vi "ProjectionExp_B.vi"() -> ()   [LabVIEW 2017]
uses:
  <instrlib>/Tektronix TDS 200 1000 2000 Series/Tektronix TDS 200 1000 2000 Series.lvlib
panel:
  in  "p":dbl
  out "Backgrond Light Intensity":dbl
  out "Units 2":string
  out "error out 3":errorcluster
  in  "Resource Name for Background":refnum<visa-resource-name>
  in  "Channel (1: Channel 1) 2":i32(ring)=1 items=["Channel 1"=1, "Channel 2"=2, "Channel 3"=3, "Channel 4"=4]
  in  "Background Light Intensity Type":i32(ring) items=["Frequency", "Mean", "Period", "Pulse Duty", "Peak to Peak", "Cycle RMS", "Minimum", "Maximum", "Rise Time", "Fall Time", "Positive Width", "Negative Width", "Amplitude", "Cycle Mean", "High", "Low", "Negative Duty", "Positive Overshoot", "Negative Overshoot", "Cursor Mean", "Burst Width", "Positive Pulse Count", "Negative Pulse Count", "Rising Edge Count", "Falling Edge Count", "Area", "Cycle Area", "RMS", "Cursor RMS"]
  in  "error in (no error) 3":errorcluster
  out "error out 2":errorcluster caption="error out"
  in  "Delay Time (s)":dbl=1.0
  in  "error in (no error) 2":errorcluster caption="error in (no error)"
  out "Iteration":i32
  out "Phi":dbl[][](array[numeric])
  out "y (Measurement \nMatrix)":dbl[][](array[numeric])
  out "VISA resource name out":refnum<visa-resource-name>
  out "Measurement":dbl
  out "Units":string
  out "error out":errorcluster
  in  "VISA resource name":refnum<visa-resource-name>
  in  "Channel (1: Channel 1)":i32(ring)=1 items=["Channel 1"=1, "Channel 2"=2, "Channel 3"=3, "Channel 4"=4]
  in  "Measurement Type (0: Frequency)":i32(ring) items=["Frequency", "Mean", "Period", "Pulse Duty", "Peak to Peak", "Cycle RMS", "Minimum", "Maximum", "Rise Time", "Fall Time", "Positive Width", "Negative Width", "Amplitude", "Cycle Mean", "High", "Low", "Negative Duty", "Positive Overshoot", "Negative Overshoot", "Cursor Mean", "Burst Width", "Positive Pulse Count", "Negative Pulse Count", "Rising Edge Count", "Falling Edge Count", "Area", "Cycle Area", "RMS", "Cursor RMS"]
  in  "error in (no error)":errorcluster
  out "Theta":dbl[][](array[numeric])
  in  "k":dbl
  in  "m":dbl
  in  "n":dbl
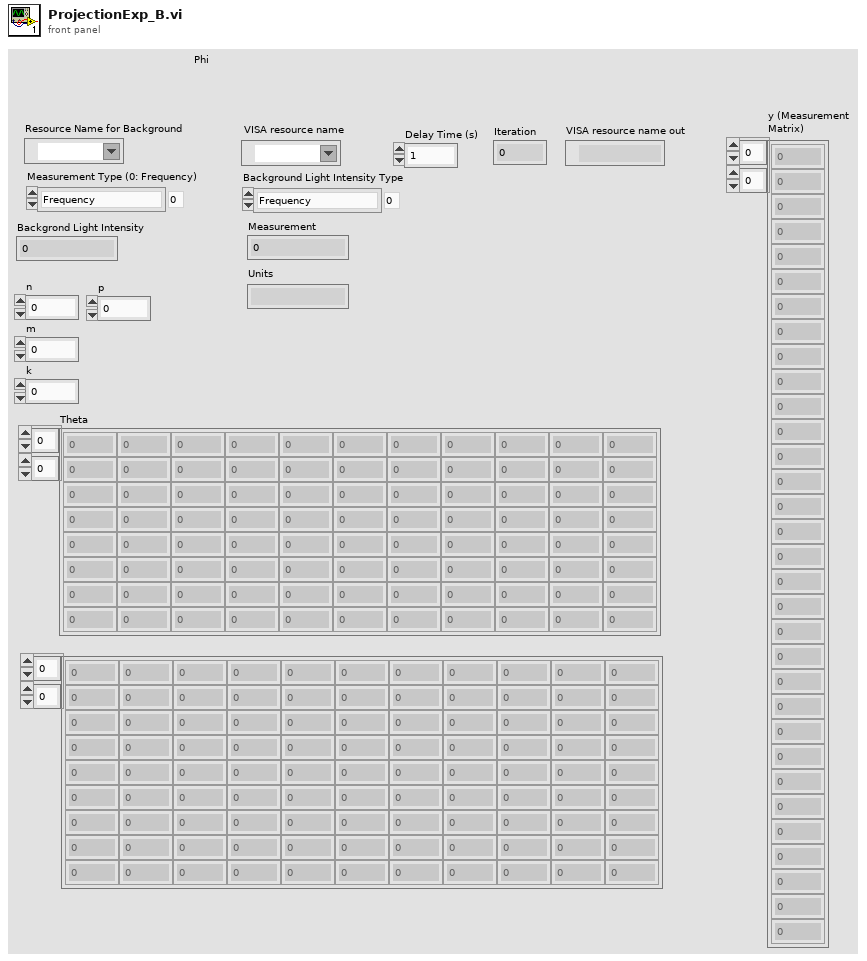
[diagram p1: front panel]
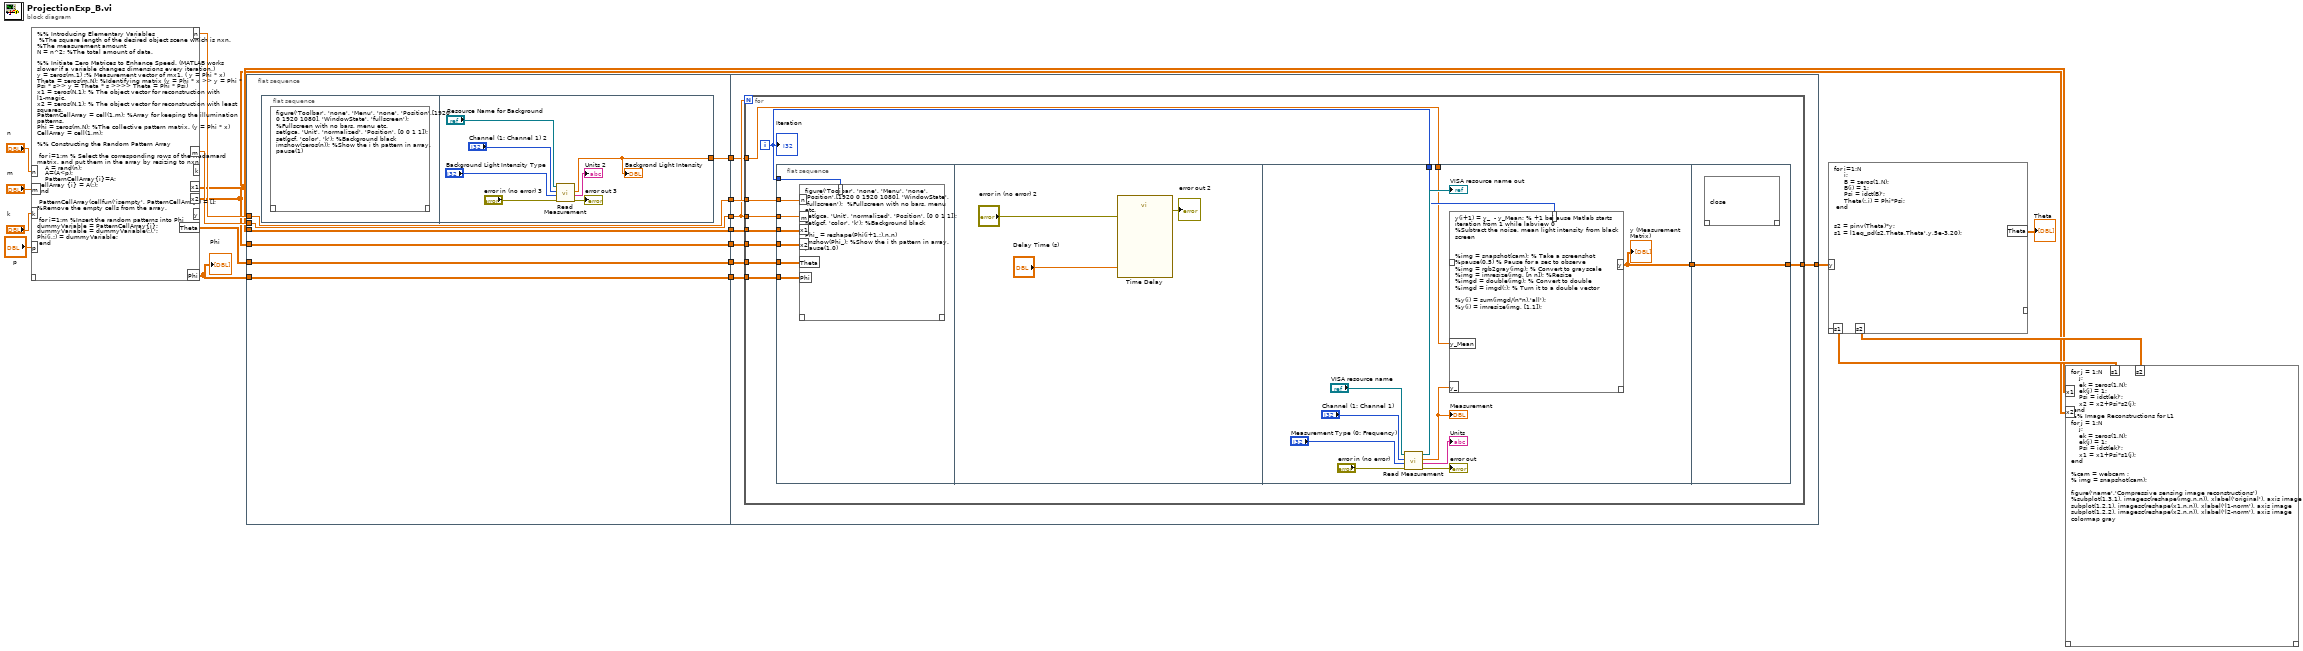
[diagram p0: block diagram]
diagram:
  n1 = script code="%% Introducing Elementary Variables\n %The square length of the desired object scene which is nxn. \n%The measurement amount\nN = n^2; %The total amount of data. \n\n%% Initiate Zero Matrices to Enhance Speed. (MATLAB works slower if a variable changes dimensions every iteration.)\ny = zeros(m,1) ;% Measurement vector of mx1. ( y = Phi * x)\nTheta = zeros(m,N); %Identifying matrix (y = Phi * x >> y = Phi * Psi * s>> y = Theta * s >>>> Theta = Phi * Psi)\nx1 = zeros(N,1); % The object vector for reconstruction with l1-magic.\nx2 = zeros(N,1); % The object vector for reconstruction with least squares.\nPatternCellArray = cell(1,m); %Array for keeping the illumination patterns.\nPhi = zeros(m,N); %The collective pattern matrix. (y = Phi * x)\nCellArray = cell(1,m);\n\n%% Constructing the Random Pattern Array\n\n for i=1:m % Select the corresponding rows of the Hadamard matrix, and put them in the array by resizing to nxn\n    A = rand(n);\n    A=(A<p);\n    PatternCellArray{i}=A;\nCellArray {i} = A(:);\nend\n \n PatternCellArray(cellfun('isempty', PatternCellArray)) = []; %Remove the empty cells from the array.\n \n for i=1:m %Insert the random patterns into Phi\ndummyVariable = PatternCellArray{i}; \ndummyVariable = dummyVariable(:).';\nPhi(i,:) = dummyVariable;\n end"("n"="n", "m"="m", "k"="k", "p"="p") -> ("n"=w14:dbl, "m"=w15:dbl, "Phi"=w10:dbl[][], "Theta"=w11:dbl[][], "x1"=w13:dbl[][], "x2"=w12:dbl[][])  [unwired: 1 in, 3 out]
  "Phi" <- w10
  n2 = flat-sequence {
    tunnel: w10 -> [w23]
    tunnel: w11 -> [w24]
    tunnel: w12 -> [w25]
    tunnel: w13 -> [w26]
    tunnel: w14 -> [w27]
    tunnel: w15 -> [w28]
    tunnel: [w28] -> w8
    tunnel: [w27] -> w7
    tunnel: [w26] -> w6
    tunnel: [w25] -> w5
    tunnel: [w24] -> w4
    tunnel: [w23] -> w3
    tunnel: [w22] -> w2
    tunnel: [w36] -> w9
    tunnel: w8 -> [w42]
    tunnel: w7 -> [w43]
    tunnel: w6 -> [w41]
    tunnel: w5 -> [w40]
    tunnel: w4 -> [w39]
    tunnel: w3 -> [w38]
    tunnel: w2 -> [w37]
    frame #0 {
      n3 = flat-sequence {
        tunnel: [w29] -> w22
        frame #0 {
          n4 = script code="figure('Toolbar', 'none', 'Menu', 'none', 'Position',[1920 0 1920 1080], 'WindowState', 'fullscreen');  %Fullscreen with no bars, menu etc.\nset(gca, 'Unit', 'normalized', 'Position', [0 0 1 1]);\nset(gcf, 'color', 'k'); %Background black\nimshow(zeros(n)); %Show the i th pattern in array. \npause(1)"() -> ()  [unwired: 1 in, 1 out]
        }
        frame #1 {
          n5 = call <instrlib>:"Read Measurement.vi"("error in (no error)"="error in (no error) 3", "Measurement Type (0: Frequency)"="Background Light Intensity Type", "Channel (1: Channel 1)"="Channel (1: Channel 1) 2", "VISA resource name"="Resource Name for Background") -> ("error out"=→"error out 3":errorcluster, "Units"=→"Units 2":string, "Measurement"=w29:dbl)  [unwired: 4 in, 1 out]
          "Backgrond Light Intensity" <- w29
        }
      }
    }
    frame #1 {
      n6 = for {
        N: w42 -> [_]
        tunnel: [w53] -> w36
        tunnel: w43 -> [w52]
        tunnel: w42 -> [w51]
        tunnel: w41 -> [w50]
        tunnel: w40 -> [w49]
        tunnel: w39 -> [w48]
        tunnel: w38 -> [w47]
        tunnel: w37 -> [w44]
        i -> [w46]
        n7 = flat-sequence {
          tunnel: w52 -> [w60]
          tunnel: w51 -> [w59]
          tunnel: w50 -> [w58]
          tunnel: w49 -> [w57]
          tunnel: w48 -> [w56]
          tunnel: w47 -> [w55]
          tunnel: w46 -> [w54]
          tunnel: w46 -> [w65]
          tunnel: [w66] -> w45
          tunnel: w44 -> [w64]
          tunnel: [w75] -> w53
          tunnel: w45 -> [w75]
          frame #0 {
            n8 = script code="figure('Toolbar', 'none', 'Menu', 'none', 'Position',[1920 0 1920 1080], 'WindowState', 'fullscreen');  %Fullscreen with no bars, menu etc.\nset(gca, 'Unit', 'normalized', 'Position', [0 0 1 1]);\nset(gcf, 'color', 'k'); %Background black\n\nPhi_ = reshape(Phi(i+1,:),n,n)\nimshow(Phi_); %Show the i th pattern in array. \npause(1.0)"("n"=w60, "m"=w59, "x1"=w58, "x2"=w57, "Theta"=w56, "Phi"=w55, "i"=w54) -> ()  [unwired: 1 in, 1 out]
          }
          frame #1 {
            n9 = call "Time Delay"("error in (no error)"="error in (no error) 2", "Delay Time (s)"="Delay Time (s)") -> ("error out"=→"error out 2":errorcluster)  [unwired: 9 in]
          }
          frame #2 {
            n10 = call <instrlib>:"Read Measurement.vi"("error in (no error)"="error in (no error)", "Measurement Type (0: Frequency)"="Measurement Type (0: Frequency)", "Channel (1: Channel 1)"="Channel (1: Channel 1)", "VISA resource name"="VISA resource name") -> ("error out"=→"error out":errorcluster, "Units"=→"Units":string, "Measurement"=w74:dbl, "VISA resource name out"=→"VISA resource name out":refnum<visa-resource-name>)  [unwired: 4 in]
            "Measurement" <- w74
            n11 = script code="y(i+1) = y_  - y_Mean; % +1 because Matlab starts iteration from 1 while labview 0 \n%Subtract the noise, mean light intensity from black screen\n\n\n%img = snapshot(cam); % Take a screenshot\n%pause(0.5) % Pause for a sec to observe\n%img = rgb2gray(img); % Convert to grayscale\n%img = imresize(img, [n n]); %Resize\n%imgd = double(img); % Convert to double \n%imgd = imgd(:); % Turn it to a double vector\n\n%y(i) = sum(imgd/(n*n),'all');\n%y(i) = imresize(img, [1,1]);"("i"=w65, "y_"=w74, "y_Mean"=w64) -> ("y"=w66:dbl[][])  [unwired: 1 in, 1 out]
            "y (Measurement \nMatrix)" <- w66
          }
          frame #3 {
            n12 = script code="close"() -> ()  [unwired: 1 in, 1 out]
          }
        }
        "Iteration" <- w46
      }
    }
  }
  n13 = script code="for i=1:N\n     i;\n     B = zeros(1,N);\n     B(i) = 1;\n     Psi = idct(B)';\n     Theta(:,i) = Phi*Psi;    \n end\n\n\ns2 = pinv(Theta)*y;\ns1 = l1eq_pd(s2,Theta,Theta',y,5e-3,20);"("y"=w9) -> ("Theta"=→"Theta":dbl[][], "s1"=w17:dbl[][], "s2"=w16:dbl[][])  [unwired: 1 in, 1 out]
  n14 = script code="for j = 1:N\n    j;\n    ek = zeros(1,N);\n    ek(j) = 1;\n    Psi = idct(ek)';\n    x2 = x2+Psi*s2(j);\n end\n%% Image Reconstructions for L1\nfor j = 1:N\n    j;\n    ek = zeros(1,N);\n    ek(j) = 1;\n    Psi = idct(ek)';\n    x1 = x1+Psi*s1(j);\nend\n\n%cam = webcam ;\n% img = snapshot(cam);\n\nfigure('name','Compressive sensing image reconstructions')\n%subplot(1,3,1), imagesc(reshape(img,n,n)), xlabel('original'), axis image\nsubplot(1,2,1), imagesc(reshape(x1,n,n)), xlabel('l1-norm'), axis image\nsubplot(1,2,2), imagesc(reshape(x2,n,n)), xlabel('l2-norm'), axis image\ncolormap gray"("s1"=w17, "s2"=w16, "x2"=w12, "x1"=w13) -> ()  [unwired: 1 in, 1 out]
